vi "API_Get Sample Data(NEW).vi"(8 "error in (no error)":errorcluster, 11 "Wait?":bool) -> (0 "error out":errorcluster, 1 "timed out?":bool, 2 "Cancelled":bool, 3 "Data Available":bool, 4 "Sample Data Array":u32[](array[numeric]), 5 "Sample No.":u32, 7 "Encoder Out":i32)   [LabVIEW 2015, in "Tool Module.lvlib"]
doc: "Retrieve the current Sample Data using the notifier created by the APi_Start Inspecting.vi. The Wait? control determines whether to simply get the last data on the notifier, or wait for a new sample. Typically use the Wait? = False to check if the inspection data has started or not. Then, use the Wait? = True when getting the sample data to display during the inpsection. This insures that each sample is new.\n\nThis vi also parses and outputs all the current data parameters, such as sample no., status, encoder plus the actual data array. The Sample data array is an array of unsigned 8-bit bytes with the following format:\n\nProbe Data:\n0: Sample Count HI Sample count is u16.\n1: Sample Count LO\n3: CD Error Code Error code from the collect data manager.\n4: Encoder byte 3 The encoder is 32-bits (4x U8).\n5: Encoder byte 2\n6: Encoder byte 1\n7: Encoder byte 0\n8: Tool status byte\n9: Probe Data... \n\nCD Error Code:\n0: Partial Array\n1: Timeout\n2: Connection Lost\n3: Other Error\n\nTool Status byte:\n0: Crash Sensor\n1: Part Present\n2: Motion\n3: Fault\n4: Inspect Switch\n5: Home\n6: Rev Limit Switch\n7: Fwd Limit Switch"
uses:
  Tool Module.lvlib
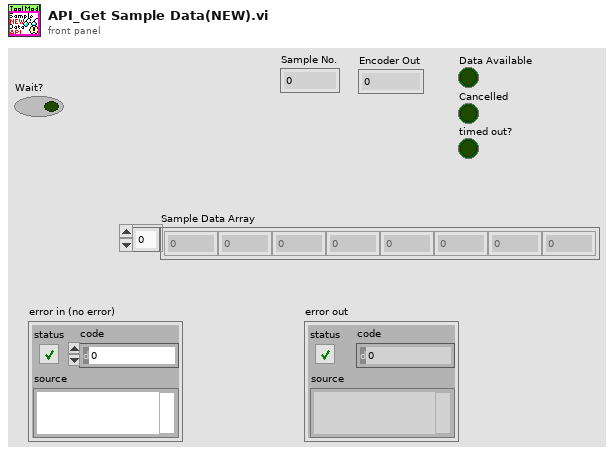
[diagram p1: front panel]
types:
  T1 = typedef "Tool Module.lvlib/_Sample Data Rtn Cluster--typedef.ctl" = cluster{"Inspecting":bool, "Acquiring Data":bool, "Success":bool, "Cancelled":bool, "Scan Data Array":u32[], "error cluster":errorcluster}
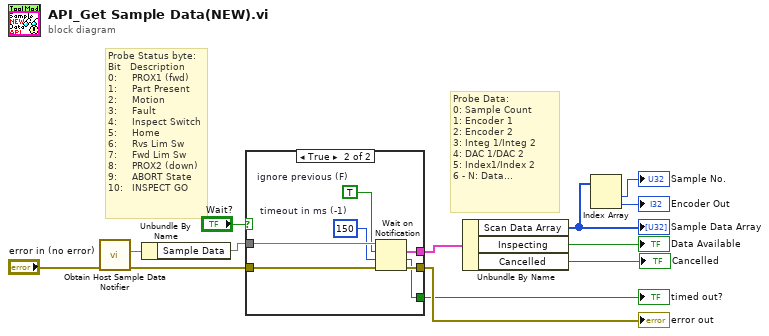
[diagram p0: block diagram]
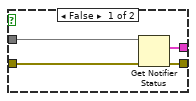
[diagram p2: hidden frame]
diagram:
  # "Probe Data:\n0: Sample Count\n1: Encoder 1\n2: Encoder 2\n3: Integ 1/Integ 2\n4: DAC 1/DAC 2\n5: Index1/Index 2\n6 - N: Data..."
  # "Probe Status byte:\nBit   Description\n0:     PROX1 (fwd)\n1:     Part Present\n2:     Motion\n3:     Fault\n4:     Inspect Switch\n5:     Home\n6:     Rvs Lim Sw\n7:     Fwd Lim Sw\n8:     PROX2 (down)\n9:     ABORT State\n10:   INSPECT GO"
  n1 = call "Obtain Host Sample Data Notifier.vi"("error in (no error)"="error in (no error)") -> ("error out"=w11:errorcluster, 2:w13)  [unwired: 8 in, 1 out]
  n2 = Unbundle By Name(w13) -> ("Sample Data"=w12)
  n3 = case shown="True" "Wait?" {
    tunnel: w12 -> [w17 w23]
    tunnel: w11 -> [w16 w24]
    tunnel: [w15 w22] -> w9
    tunnel: [w14 w21] -> w7
    tunnel: [_ w18] -> w5
    frame False {
      n4 = Get Notifier Status(notifier=w17, error in (no error)=w16) -> (current notification=w14:T1, error out=w15:errorcluster)  [unwired: 3 out]
    }
    frame True {
      w19 = TRUE  # ignore previous (F)
      w20 = 150  # timeout in ms (-1)
      n5 = Wait on Notification(notifier=w23, ignore previous (F)=w19, timeout in ms (-1)=w20, error in (no error)=w24) -> (notification=w21:T1, timed out?=w18:bool, error out=w22:errorcluster)  [unwired: 1 out]
    }
  }
  "error out" <- w9
  "timed out?" <- w5
  n6 = Unbundle By Name(w7) -> ("Scan Data Array"=w4:u32[], "Inspecting"=→"Data Available":bool, "Cancelled"=→"Cancelled":bool)
  "Sample Data Array" <- w4
  n7 = Index Array(array=w4) -> (element #1=→"Sample No.":u32, element #2=→"Encoder Out":u32)  [unwired: 2 in]
